vi "Remove Key.vi"(7 "section":string, 8 "error in (no error)":errorcluster, 10 "key":string, 11 "refnum":T1) -> (0 "error out":errorcluster, 2 "found?":bool, 3 "refnum out":T1)   [LabVIEW 2010, in "NI_LVConfig.lvlib"]
doc: "Removes a <B>key</B> in a specified section from the configuration data identified by <B>refnum</B>."
uses:
  NI_LVConfig.lvlib
  Config Data RefNum.ctl
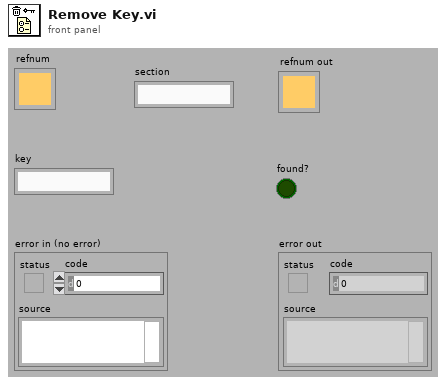
[diagram p1: front panel]
types:
  T1 = typedef "NI_LVConfig.lvlib/Config Data RefNum.ctl" = refnum<k1>
  T2 = typedef "NI_LVConfig.lvlib/Config Queue.ctl" = refnum<queue>
  T3 = typedef "NI_LVConfig.lvlib/Config Data.ctl" = cluster{"sections":T4[], "path":path, "dirty":bool}
  T4 = typedef "NI_LVConfig.lvlib/Section.ctl" = cluster{"name":string, "comment":string, "kvc":string[][]}
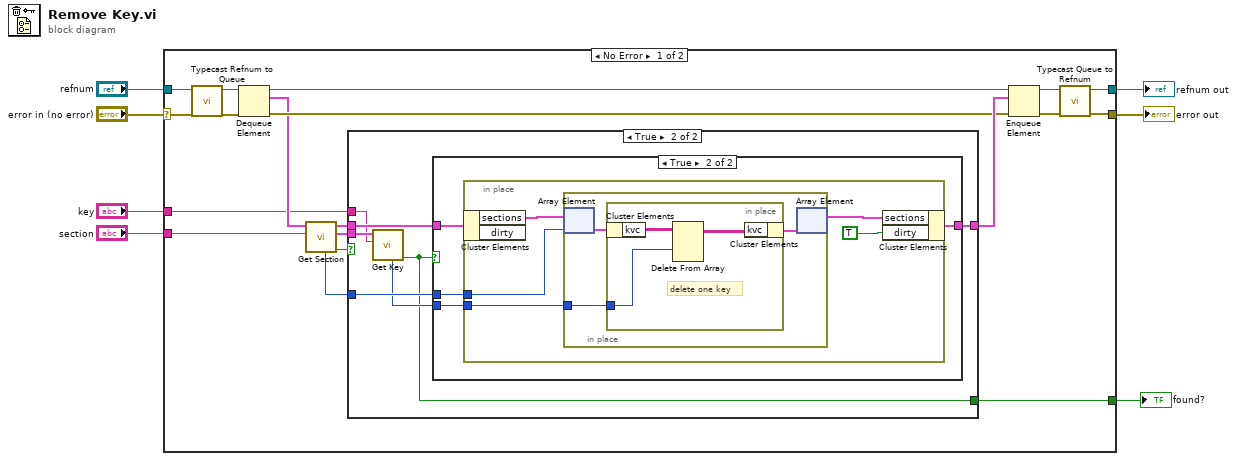
[diagram p0: block diagram]
diagram:
  n1 = case shown="No Error" "error in (no error)" {
    selector: "error in (no error)" -> [w8 w50]
    tunnel: [w21 w50] -> w1
    tunnel: [w18 w49] -> w3
    tunnel: "refnum" -> [w20 w49]
    tunnel: "section" -> [w9 _]
    tunnel: "key" -> [w15 _]
    tunnel: [w10 _] -> w2
    frame No Error {
      n2 = call "Typecast Refnum to Queue.vi"("refnum in"=w20) -> ("queue out"=w17:T2)  [unwired: 10 out]
      n3 = Dequeue Element(queue=w17, error in (no error)=w8) -> (queue out=w23:T2, element=w16:T3, error out=w22:errorcluster)  [unwired: 2 out]
      n4 = call "Get Section.vi"("section"=w9, "element"=w16) -> ("section exists?"=w12:bool, "section data"=w14:T4, "element out"=w13:T3, "section index"=w11:i32)  [unwired: 2 in, 4 out]
      n5 = case shown="True" w12 {
        tunnel: [w25 w32] -> w24
        tunnel: w15 -> [_ w26]
        tunnel: w14 -> [_ w31]
        tunnel: w13 -> [w25 w30]
        tunnel: w11 -> [_ w29]
        tunnel: [_ w27] -> w10
        frame False {
        }
        frame True {
          n6 = call "Get Key.vi"("key"=w26, "section data"=w31) -> ("key exists?"=w27:bool, "key index"=w28:i32)  [unwired: 3 in, 5 out]
          n7 = case shown="True" w27 {
            tunnel: w29 -> [_ w36]
            tunnel: w28 -> [_ w35]
            tunnel: [w33 w34] -> w32
            tunnel: w30 -> [w33 w37]
            frame False {
            }
            frame True {
              n8 = in-place "In Place Element Structure" {
                in-place-border: w36 -> [w41]
                in-place-border: w35 -> [w40]
                n9 = in-place-cluster #1(w37) -> ("sections"=w42:T4[])  [unwired: 1 out]
                n10 = in-place "In Place Element Structure" {
                  in-place-border: w40 -> [w44]
                  n11 = in-place-array #2(w42, w41) -> (w45:T4)
                  n12 = in-place "In Place Element Structure" {
                    in-place-border: w44 -> [w46]
                    # "delete one key"
                    n13 = in-place-cluster #3(w45) -> ("kvc"=w48:string[][])
                    n14 = Delete From Array(array=w48, index (row)=w46) -> (array with subset deleted=w47:string[][])  [unwired: 2 in, 1 out]
                    n15 = in-place-cluster #3("kvc"=w47) -> (w43:T4)
                  }
                  n16 = in-place-array #2(w43) -> (w39:T4[])  [unwired: 1 out]
                }
                n17 = in-place-cluster #1("sections"=w39, "dirty"=TRUE) -> (w34:T3)
              }
            }
          }
        }
      }
      n18 = Enqueue Element(queue=w23, element=w24, error in (no error)=w22) -> (queue out=w19:T2, error out=w21:errorcluster)  [unwired: 2 out]
      n19 = call "Typecast Queue to Refnum.vi"("queue in"=w19) -> ("refnum out"=w18:T1)  [unwired: 10 out]
    }
    frame Error {
    }
  }
  "error out" <- w1
  "found?" <- w2
  "refnum out" <- w3
